vi "GetDTCMap.vi"(0 "Server":string, 1 "Sequence Context In":refnum<k7>, 3 "Username":string, 5 "error in (no error)":errorcluster, 9 "ParamType":string, 11 "subMachine":string, 12 "MechID":string) -> (4 "Initial":u32[](array[numeric]), 6 "Final":u32[](array[numeric]), 8 "Status":dbl[](array[numeric]), 10 "Map_Defs":string[](array[string]), 14 "output cluster":cluster{string[], i32[]}, 15 "error out":errorcluster)   [LabVIEW 2017]
uses:
  C:/Projects/DTC/HVL4/SEL/v11-06/SEL 2/vi/DTC_Memory_Map/Sensata.MES.Integration.ST.ParameterControl.dll
  SEL 2/vi/DTC_Memory_Map/Sensata.MES.Integration.ST.ParameterControl.dll
panel:
  out "GetParameterSetJSON":string
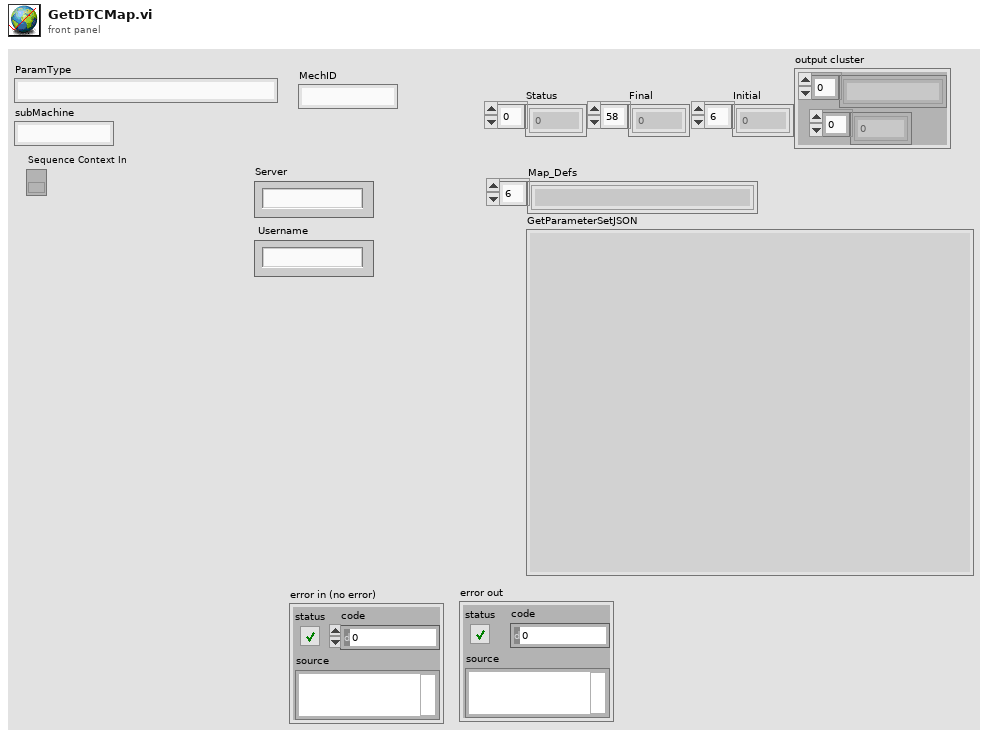
[diagram p1: front panel]
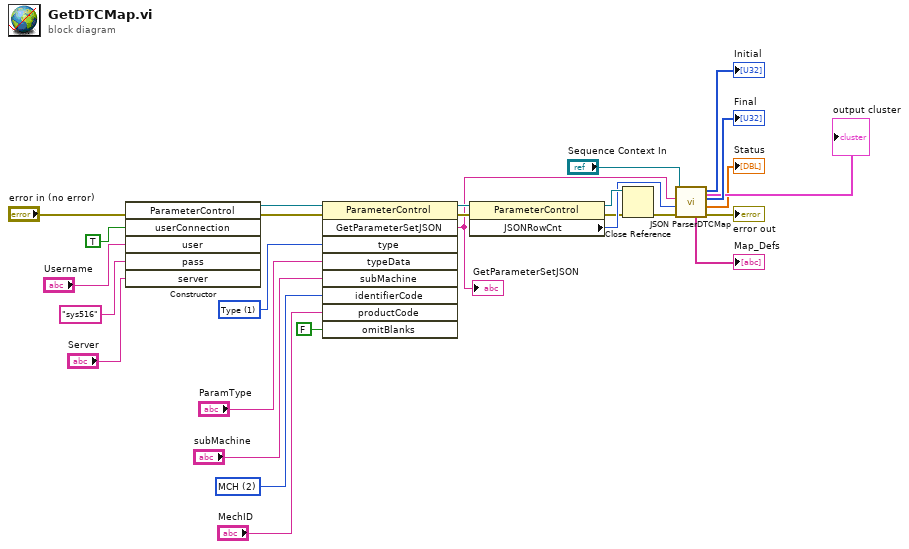
[diagram p0: block diagram]
diagram:
  w21 = 2 items=["BOM", "SMT", "MCH"] ("identifierCode")
  w24 = 1 items=["Process", "Type"] ("type")
  n1 = constructor class="ParameterControl"(error in="error in (no error)", "userConnection"=TRUE, "user"="Username", "pass"="sys516", "server"="Server") -> (reference out=w26:refnum<k24>, error out=w25:errorcluster)  [unwired: 2 in, 5 out]
  n2 = invoke class="ParameterControl" method="GetParameterSetJSON"(reference=w26, error in=w25, "type"=w24, "typeData"="ParamType", "subMachine"="subMachine", "identifierCode"=w21, "productCode"="MechID", "omitBlanks"=FALSE) -> (reference out=w18:refnum<k24>, error out=w17:errorcluster, "GetParameterSetJSON"=w14:string)  [unwired: 1 in, 6 out]
  "GetParameterSetJSON" <- w14
  n3 = property class="ParameterControl"(reference=w18, error in=w17) -> (reference out=w16:refnum<k24>, error out=w12:errorcluster, "JSONRowCnt"=w13:i32)
  n4 = Close Reference(reference=w16, error in (no error)=w12) -> (error out=w8:errorcluster)
  n5 = call "JSON ParserDTCMap.vi"("Error In"=w8, "NumElements"=w13, "jsonin"=w14, "Sequence Context In"="Sequence Context In") -> ("error out"=→"error out":errorcluster, "Status"=→"Status":dbl[], "Final"=→"Final":u32[], "Initial"=→"Initial":u32[], "Map_Defs"=→"Map_Defs":string[], "output cluster"=→"output cluster":cluster{string[], i32[]})  [unwired: 2 in]
